vi "Delete All DMA Blocks.vi"(8 "error in (no error)":errorcluster, 11 "Device Ref In":T1=18446744073709551615 format="%.0x") -> (0 "error out":errorcluster, 3 "Device Ref Out":T1=18446744073709551615 format="%.0x")   [LabVIEW 2017, in "GE_RM_System Explorer.lvlib"]
uses:
  GE_RM_System Explorer.lvlib
  <vilib>/NI Veristand/Custom Device API/Custom Device Item Ref.ctl
  Shared/Global.vi
  <vilib>/NI VeriStand/Custom Device API/Custom Device API.lvlib
  Shared/GE_RM_Shared.lvlib
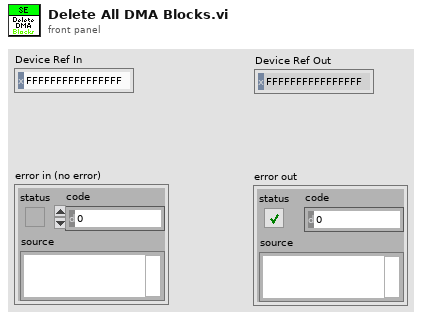
[diagram p1: front panel]
types:
  T1 = typedef "Custom Device API.lvlib/Custom Device Item Ref.ctl" = u64
  T2 = typedef "Custom Device API.lvlib/Custom Device Item Info.ctl" = cluster{"Name":string, "Is Channel":bool, "GUID":string, "Is Waveform":bool}
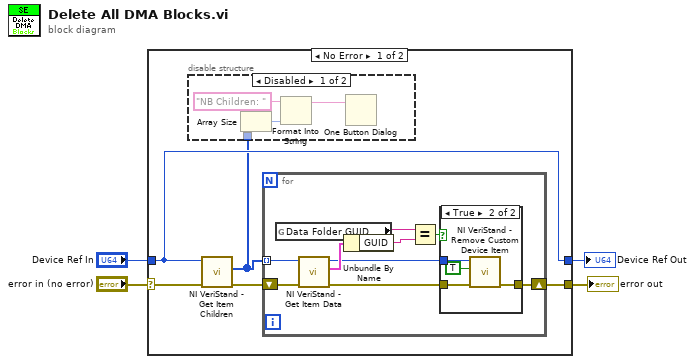
[diagram p0: block diagram]
diagram:
  n1 = case shown="No Error" "error in (no error)" {
    selector: "error in (no error)" -> [w8 w28]
    tunnel: "Device Ref In" -> [w6 w29]
    tunnel: [w9 w28] -> w3
    tunnel: [w6 w29] -> w1
    frame No Error {
      n2 = call <vilib>:"NI VeriStand - Get Item Children.vi"("error in (no error)"=w8, "Item Ref in"=w6) -> ("error out"=w7:errorcluster, "Child Refs"=w5:T1[])  [unwired: 6 in, 2 out]
      n3 = disable-structure shown="Disabled" {
        disable-tunnel: w5 -> [w10 _]
        frame Disabled {
          n4 = Array Size(array=w10) -> (size(s)=w13:i32)
          n5 = Format Into String(initial string="NB Children: ", w13) -> (resulting string=w12:string)  [unwired: 2 in, 1 out]
          n6 = One Button Dialog(message=w12) -> ()  [unwired: 1 in, 1 out]
        }
        frame Enabled {
        }
      }
      n7 = for {
        shift-right: [w16] -> w9
        shift-left: w7 -> [w22]
        tunnel: w5 -> [w21] mode=indexing
        n8 = global read "Global.vi" "Data Folder GUID"() -> (w18:string)
        n9 = call <vilib>:"NI VeriStand - Get Item Data.vi"("error in (no error)"=w22, "Item Ref in"=w21) -> ("error out"=w17:errorcluster, "Item Info"=w20:T2, "Item Ref out"=w14:T1)  [unwired: 6 in, 1 out]
        n10 = Unbundle By Name(w20) -> ("GUID"=w19:string)
        n11 = Equal?(x=w18, y=w19) -> (x = y?=w15:bool)
        n12 = case shown="True" w15 {
          tunnel: w17 -> [w23 w27]
          tunnel: [w23 w26] -> w16
          tunnel: w14 -> [_ w24]
          frame False {
          }
          frame True {
            n13 = call <vilib>:"NI VeriStand - Remove Custom Device Item.vi"("error in (no error)"=w27, "Force Delete (F)"=TRUE, "Item Ref in"=w24) -> ("error out"=w26:errorcluster)  [unwired: 7 in, 1 out]
          }
        }
      }
    }
    frame Error {
    }
  }
  "error out" <- w3
  "Device Ref Out" <- w1
